vi "Initialize Actor.vi"(7 "Host Name":string, 8 "error in (no error)":errorcluster, 9 "Actor Name":string, 10 "Message Broker Interface":refnum<class "Message Broker Interface.lvclass">, 11 "User Interface in":refnum<class "User Interface.lvclass">) -> (0 "error out":errorcluster, 3 "User Interface out":refnum<class "User Interface.lvclass">)   [LabVIEW 2016, in "CLD Exam - ATM.lvlib" / "User Interface.lvclass"]
uses:
  User Interface.lvclass
  Mediator/Classes/Message Broker Interface/Message Broker Interface.lvclass
  User Interface.lvclass/User Interface.ctl
  Mediator/Classes/Message Transport Event/Message Transport Event.lvclass
  D:/Repos/Stream/software/Mediator/Classes/Message Transport Interface/Message Transport Interface.lvclass
  Mediator/Classes/Mediated Synchronous Actor/Mediated Synchronous Actor.lvclass
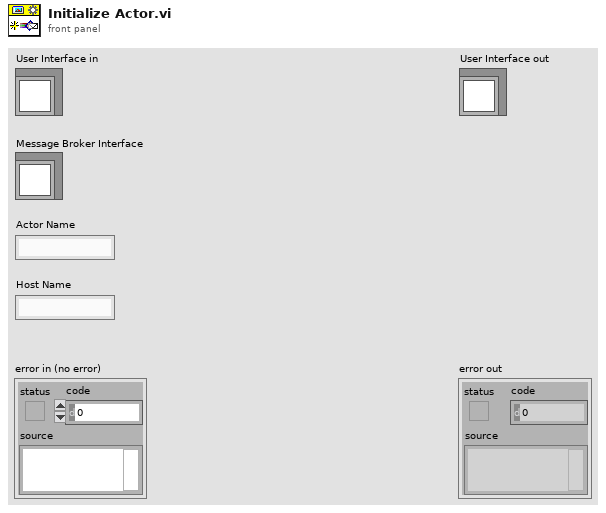
[diagram p1: front panel]
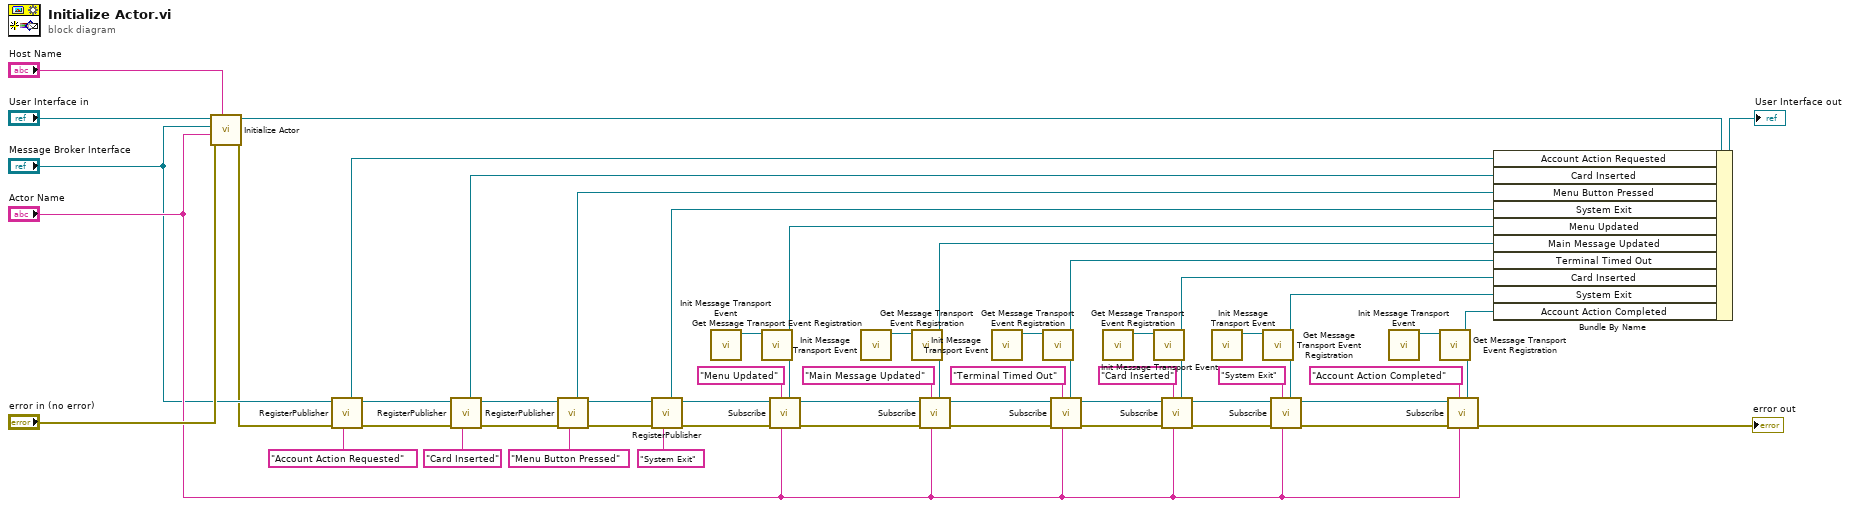
[diagram p0: block diagram]
diagram:
  n1 = call-parent "Initialize Actor.vi"("Host Name"="Host Name", "error in (no error)"="error in (no error)", "Actor Name"="Actor Name", "Message Broker Interface"="Message Broker Interface", "Mediated Synchronous Actor in"="User Interface in") -> ("error out"=w5:errorcluster, "Mediated Synchronous Actor out"=w56:refnum<class "User Interface.lvclass">)  [unwired: 5 in]
  n2 = call-dynamic "RegisterPublisher.vi"("Topic Name"="Account Action Requested", "error in (no error)"=w5, "Message Broker Interface in"="Message Broker Interface") -> ("error out"=w4:errorcluster, "Message Broker Interface out"=w6:refnum<class "Message Broker Interface.lvclass">, "Transport"=w3:refnum<class "Message Transport Queue.lvclass">)  [unwired: 4 in, 2 out]
  n3 = call-dynamic "RegisterPublisher.vi"("Topic Name"="Card Inserted", "error in (no error)"=w4, "Message Broker Interface in"=w6) -> ("error out"=w51:errorcluster, "Message Broker Interface out"=w50:refnum<class "Message Broker Interface.lvclass">, "Transport"=w53:refnum<class "Message Transport Queue.lvclass">)  [unwired: 4 in, 2 out]
  n4 = call-dynamic "RegisterPublisher.vi"("Topic Name"="Menu Button Pressed", "error in (no error)"=w51, "Message Broker Interface in"=w50) -> ("error out"=w1:errorcluster, "Message Broker Interface out"=w2:refnum<class "Message Broker Interface.lvclass">, "Transport"=w49:refnum<class "Message Transport Queue.lvclass">)  [unwired: 4 in, 2 out]
  n5 = call-dynamic "RegisterPublisher.vi"("Topic Name"="System Exit", "error in (no error)"=w1, "Message Broker Interface in"=w2) -> ("error out"=w44:errorcluster, "Message Broker Interface out"=w45:refnum<class "Message Broker Interface.lvclass">, "Transport"=w47:refnum<class "Message Transport Queue.lvclass">)  [unwired: 4 in, 2 out]
  n6 = call "Init Message Transport Event.vi"() -> ("Message Transport Event out"=w46:refnum<class "Message Transport Event.lvclass">)  [unwired: 10 in, 1 out]
  n7 = call "Get Message Transport Event Registration.vi"("Message Transport Event in"=w46) -> ("Event Registration Refnum"=w41:refnum<event-registration>, "Message Transport Event out"=w43:refnum<class "Message Transport Event.lvclass">)  [unwired: 7 in, 2 out]
  n8 = call-dynamic "Subscribe.vi"("Message Transport Interface"=w43, "Subscriber Name"="Actor Name", "Topic Name"="Menu Updated", "error in (no error)"=w44, "Message Broker Interface in"=w45) -> ("error out"=w17:errorcluster, "Message Broker Interface out"=w18:refnum<class "Message Broker Interface.lvclass">)  [unwired: 4 in, 1 out]
  n9 = call "Init Message Transport Event.vi"() -> ("Message Transport Event out"=w23:refnum<class "Message Transport Event.lvclass">)  [unwired: 10 in, 1 out]
  n10 = call "Get Message Transport Event Registration.vi"("Message Transport Event in"=w23) -> ("Event Registration Refnum"=w22:refnum<event-registration>, "Message Transport Event out"=w24:refnum<class "Message Transport Event.lvclass">)  [unwired: 7 in, 2 out]
  n11 = call-dynamic "Subscribe.vi"("Message Transport Interface"=w24, "Subscriber Name"="Actor Name", "Topic Name"="Main Message Updated", "error in (no error)"=w17, "Message Broker Interface in"=w18) -> ("error out"=w40:errorcluster, "Message Broker Interface out"=w39:refnum<class "Message Broker Interface.lvclass">)  [unwired: 4 in, 1 out]
  n12 = call "Init Message Transport Event.vi"() -> ("Message Transport Event out"=w38:refnum<class "Message Transport Event.lvclass">)  [unwired: 10 in, 1 out]
  n13 = call "Get Message Transport Event Registration.vi"("Message Transport Event in"=w38) -> ("Event Registration Refnum"=w21:refnum<event-registration>, "Message Transport Event out"=w37:refnum<class "Message Transport Event.lvclass">)  [unwired: 7 in, 2 out]
  n14 = call-dynamic "Subscribe.vi"("Message Transport Interface"=w37, "Subscriber Name"="Actor Name", "Topic Name"="Terminal Timed Out", "error in (no error)"=w40, "Message Broker Interface in"=w39) -> ("error out"=w31:errorcluster, "Message Broker Interface out"=w32:refnum<class "Message Broker Interface.lvclass">)  [unwired: 4 in, 1 out]
  n15 = call "Init Message Transport Event.vi"() -> ("Message Transport Event out"=w33:refnum<class "Message Transport Event.lvclass">)  [unwired: 10 in, 1 out]
  n16 = call "Get Message Transport Event Registration.vi"("Message Transport Event in"=w33) -> ("Event Registration Refnum"=w20:refnum<event-registration>, "Message Transport Event out"=w34:refnum<class "Message Transport Event.lvclass">)  [unwired: 7 in, 2 out]
  n17 = call-dynamic "Subscribe.vi"("Message Transport Interface"=w34, "Subscriber Name"="Actor Name", "Topic Name"="Card Inserted", "error in (no error)"=w31, "Message Broker Interface in"=w32) -> ("error out"=w26:errorcluster, "Message Broker Interface out"=w27:refnum<class "Message Broker Interface.lvclass">)  [unwired: 4 in, 1 out]
  n18 = call "Init Message Transport Event.vi"() -> ("Message Transport Event out"=w30:refnum<class "Message Transport Event.lvclass">)  [unwired: 10 in, 1 out]
  n19 = call "Get Message Transport Event Registration.vi"("Message Transport Event in"=w30) -> ("Event Registration Refnum"=w19:refnum<event-registration>, "Message Transport Event out"=w29:refnum<class "Message Transport Event.lvclass">)  [unwired: 7 in, 2 out]
  n20 = call-dynamic "Subscribe.vi"("Message Transport Interface"=w29, "Subscriber Name"="Actor Name", "Topic Name"="System Exit", "error in (no error)"=w26, "Message Broker Interface in"=w27) -> ("error out"=w13:errorcluster, "Message Broker Interface out"=w14:refnum<class "Message Broker Interface.lvclass">)  [unwired: 4 in, 1 out]
  n21 = call "Init Message Transport Event.vi"() -> ("Message Transport Event out"=w9:refnum<class "Message Transport Event.lvclass">)  [unwired: 10 in, 1 out]
  n22 = call "Get Message Transport Event Registration.vi"("Message Transport Event in"=w9) -> ("Event Registration Refnum"=w10:refnum<event-registration>, "Message Transport Event out"=w15:refnum<class "Message Transport Event.lvclass">)  [unwired: 7 in, 2 out]
  n23 = call-dynamic "Subscribe.vi"("Message Transport Interface"=w15, "Subscriber Name"="Actor Name", "Topic Name"="Account Action Completed", "error in (no error)"=w13, "Message Broker Interface in"=w14) -> ("error out"=→"error out":errorcluster)  [unwired: 4 in, 2 out]
  n24 = Bundle By Name(cluster=w56, "Account Action Requested"=w3, "Card Inserted"=w53, "Menu Button Pressed"=w49, "System Exit"=w47, "Menu Updated"=w41, "Main Message Updated"=w22, "Terminal Timed Out"=w21, "Card Inserted"=w20, "System Exit"=w19, "Account Action Completed"=w10) -> (→"User Interface out":refnum<class "User Interface.lvclass">)
